vi "Increment.vi"(11 "Number":i32) -> (3 "Result":i32)   [LabVIEW 2021]
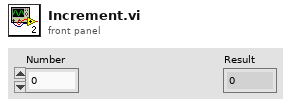
[diagram p1: front panel]
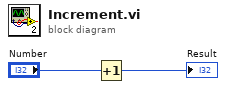
[diagram p0: block diagram]
diagram:
  n1 = Increment(x="Number") -> (x+1=→"Result":i32)
